vi "PH_AxisGUI_BaseClass.PC Reset.vi"(0 "i ref in":refnum<vi>, 2 "Addresses":T1[](array[typedef]), 5 "error in":errorcluster) -> (14 "i ref out":refnum<vi>, 19 "error out":errorcluster)   [LabVIEW 2014, in "PH_AxisGUI_BaseClass.lvlib"]
doc: "This VI acts on several axes."
uses:
  PH_AxisGUI_BaseClass.lvlib
  PH_Stepmotor_BaseClass/PH_Stepmotor_BaseClass.Axis Address.ctl
  PH_Stepmotor_BaseClass/PH_Stepmotor_BaseClass.lvlib
  CSCore/CSSystem/CSSystemLib/CSSystemLib.lvlib
  PH_Common/PH_Common.lvlib
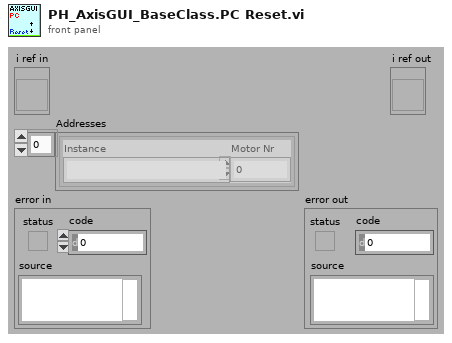
[diagram p1: front panel]
types:
  T1 = typedef "PH_Stepmotor_BaseClass.lvlib/PH_Stepmotor_BaseClass.Axis Address.ctl" = cluster{"Instance":string, "Motor Nr":i32}
  T2 = cluster{"Address":T1, "GUI Class":string, "GUI Instance":string}[]
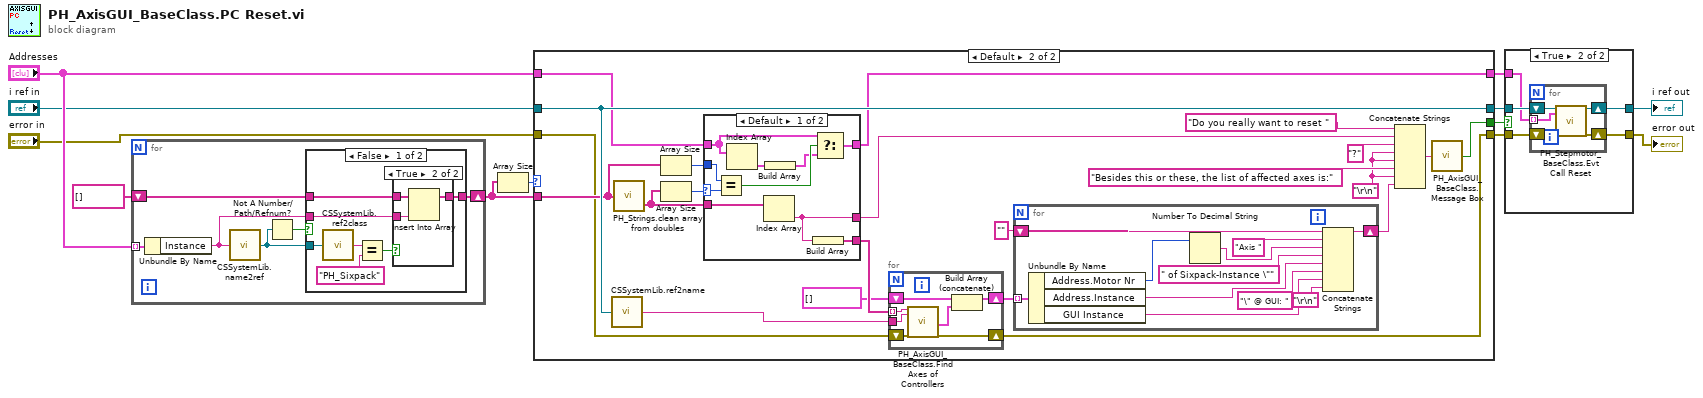
[diagram p0: block diagram]
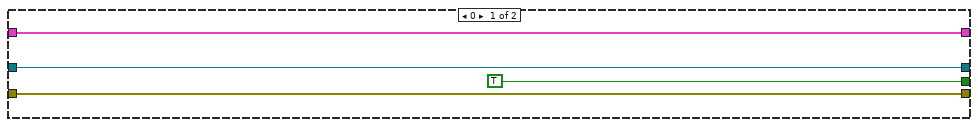
[diagram p2: hidden frame]
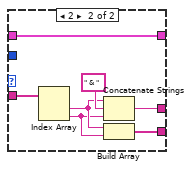
[diagram p3: hidden frame]
diagram:
  n1 = for {
    tunnel: "Addresses" -> [w17] mode=indexing
    shift-right: [w18] -> w9
    shift-left: string[] [] -> [w16]
    n2 = Unbundle By Name(w17) -> ("Instance"=w15:string)
    n3 = call "CSSystemLib.name2ref.vi"("name"=w15) -> ("obj refnum"=w13:refnum<vi>)
    n4 = Not A Number/Path/Refnum?(number/path/refnum=w13) -> (NaN/Path/Refnum?=w14:bool)
    n5 = case shown="False" w14 {
      tunnel: [w25 w30] -> w18
      tunnel: w15 -> [w24 _]
      tunnel: w16 -> [w23 w30]
      tunnel: w13 -> [w21 _]
      frame False {
        n6 = call "CSSystemLib.ref2class.vi"("obj refnum"=w21) -> ("class"=w20:string)
        n7 = Equal?(x=w20, y="PH_Sixpack") -> (x = y?=w19:bool)
        n8 = case shown="True" w19 {
          tunnel: [w26 w29] -> w25
          tunnel: w24 -> [_ w28]
          tunnel: w23 -> [w26 w27]
          frame False {
          }
          frame True {
            n9 = Insert Into Array(array=w27, new element=w28) -> (w29:string[])  [unwired: 1 in]
          }
        }
      }
      frame True {
      }
    }
  }
  n10 = Array Size(array=w9) -> (size(s)=w10:i32)
  n11 = case shown="Default" w10 {
    tunnel: [TRUE ("OK?") w56] -> w6
    tunnel: [w32 w37] -> w7
    tunnel: "error in" -> [w32 w40]
    tunnel: "i ref in" -> [w33 w45]
    tunnel: w9 -> [_ w42]
    tunnel: "Addresses" -> [w34 w44]
    tunnel: [w34 w43] -> w11
    tunnel: [w33 w45] -> w12
    frame 0 {
    }
    frame Default {
      w52 = "\r\n"
      n12 = call "CSSystemLib.ref2name.vi"("obj refnum"=w45) -> ("name"=w38:string)
      n13 = call "PH_Strings.clean array from doubles.vi"("Array Input"=w42) -> ("Cleaned Array Output"=w46:string[])  [unwired: 1 out]
      n14 = Array Size(array=w42) -> (size(s)=w41:i32)
      n15 = Array Size(array=w46) -> (size(s)=w47:i32)
      n16 = case shown="Default" w47 {
        selector: w47 -> [w80 _]
        tunnel: w46 -> [w84 w90]
        tunnel: [w82 w87] -> w50
        tunnel: [w83 w86] -> w39
        tunnel: w44 -> [w77 w85]
        tunnel: [w79 w85] -> w43
        tunnel: w41 -> [w81 _]
        frame Default {
          n17 = Equal?(x=w81, y=w80) -> (x = y?=w78:bool)
          n18 = Index Array(array=w77) -> (element=w76:T1)  [unwired: 1 in]
          n19 = Index Array(array=w84) -> (element=w82:string)  [unwired: 1 in]
          n20 = Build Array(w76) -> (w75:T1[])
          n21 = Build Array(w82) -> (w83:string[])
          n22 = Select(t=w77, s=w78, f=w75) -> (s? t:f=w79:T1[])
        }
        frame 2 {
          n23 = Index Array(array=w90) -> (element #1=w89:string, element #2=w88:string)  [unwired: 2 in]
          n24 = Concatenate Strings(w89, " & " ("string"), w88) -> (w87:string)
          n25 = Build Array(w89, w88) -> (w86:string[])
        }
      }
      n26 = for {
        tunnel: w38 -> [w73]
        tunnel: w39 -> [w74] mode=indexing
        shift-right: [w71] -> w37
        shift-left: w40 -> [w72]
        shift-right: [w69] -> w36
        shift-left: T2 [] ("Result") -> [w68]
        n27 = call "PH_AxisGUI_BaseClass.Find Axes of Controllers.vi"("Own Motion Instance (N/A)"=w74, "GUI Instance (N/A)"=w73, "error in"=w72) -> ("Result"=w70:T2, "error out"=w71:errorcluster)  [unwired: 15 in]
        n28 = Build Array (concatenate)(w68, w70) -> (w69:T2)
      }
      n29 = for {
        shift-right: [w66] -> w48
        shift-left: "" -> [w64]
        tunnel: w36 -> [w61] mode=indexing
        n30 = Unbundle By Name(w61) -> ("Address.Motor Nr"=w58:i32, "Address.Instance"=w59:string, "GUI Instance"=w60:string)
        n31 = Number To Decimal String(number=w58) -> (decimal integer string=w57:string)  [unwired: 1 in]
        n32 = Concatenate Strings(w64, "Axis " ("string"), w57, " of Sixpack-Instance \"" ("string"), w59, "\" @ GUI: " ("string"), w60, "\r\n") -> (w66:string)
      }
      n33 = Concatenate Strings("Do you really want to reset ", w50, "?", w52, w52, "Besides this or these, the list of affected axes is:" ("string"), w52, w48) -> (w51:string)
      n34 = call "PH_AxisGUI_BaseClass.Message Box.vi"("String"=w51) -> ("OK?"=w56:bool)
    }
  }
  n35 = case shown="True" w6 {
    tunnel: [w93 w98] -> w2
    tunnel: [w92 w97] -> w1
    tunnel: w12 -> [w93 w96]
    tunnel: w7 -> [w92 w95]
    tunnel: w11 -> [_ w94]
    frame False {
    }
    frame True {
      n36 = for {
        shift-right: [w102] -> w97
        shift-left: w95 -> [w100]
        shift-right: [w103] -> w98
        shift-left: w96 -> [w101]
        tunnel: w94 -> [w99] mode=indexing
        n37 = call "PH_Stepmotor_BaseClass.Evt Call Reset.vi"("i ref in"=w101, "Address"=w99, "error in"=w100) -> ("i ref out"=w103:refnum<vi>, "error out"=w102:errorcluster)  [unwired: 15 in]
      }
    }
  }
  "error out" <- w1
  "i ref out" <- w2
